vi "AutoShootRear.vi"() -> ()   [LabVIEW 2015]
uses:
  Typedef/IntakeControllerActions.ctl
  Typedef/IntakeControllerMsg.ctl
  ArmController/ArmController.lvlib
panel:
  in  "milliseconds to wait":u32=600
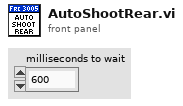
[diagram p1: front panel]
types:
  T1 = typedef "IntakeControllerMsg.ctl" = cluster{"Cmd":T2, "Data":variant}
  T2 = typedef "IntakeControllerActions.ctl" = enum16{"Wait on Intake Rear", "Wait on Angle Rear", "Go To Angle Rear", "Wait on Intake Front", "Wait on Angle Front", "Set Roller Front", "Set Roller Rear", "Go To Angle Front", "Wait ms"}
  T3 = cluster{"Down":dbl, "Pickup":dbl, "Shoot":dbl, "Turtle":dbl, "Intake Block":dbl, "Intake Transfer":dbl}
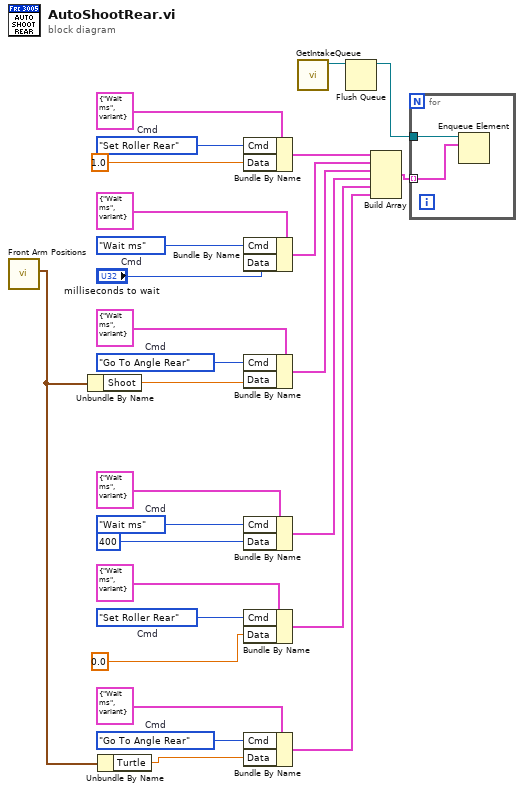
[diagram p0: block diagram]
diagram:
  w28 = IntakeControllerActions."Go To Angle Rear"  # Cmd
  w19 = IntakeControllerActions."Set Roller Rear"  # Cmd
  w23 = IntakeControllerActions."Wait ms"  # Cmd
  w16 = IntakeControllerActions."Go To Angle Rear"  # Cmd
  w11 = IntakeControllerActions."Wait ms"  # Cmd
  w8 = IntakeControllerActions."Set Roller Rear"  # Cmd
  n1 = call "Front Arm Positions.vi"() -> ("Rear Arm"=w1:T3)  [unwired: 10 in, 1 out]
  n2 = Unbundle By Name(w1) -> ("Shoot"=w2:dbl)
  n3 = Unbundle By Name(w1) -> ("Turtle"=w3:dbl)
  n4 = Bundle By Name(cluster=T1 {"Cmd"=enum."Wait ms", "Data"=variant(i32 50)} ("output cluster"), "Cmd"=w8, "Data"=1.0 ("Diffs")) -> (w10:T1)
  n5 = Bundle By Name(cluster=T1 {"Cmd"=enum."Wait ms", "Data"=variant(i32 50)} ("output cluster"), "Cmd"=w11, "Data"="milliseconds to wait") -> (w14:T1)
  n6 = Bundle By Name(cluster=T1 {"Cmd"=enum."Wait ms", "Data"=variant(i32 50)} ("output cluster"), "Cmd"=w16, "Data"=w2) -> (w17:T1)
  n7 = Bundle By Name(cluster=T1 {"Cmd"=enum."Wait ms", "Data"=variant(i32 50)} ("output cluster"), "Cmd"=w23, "Data"=u32 400 ("milliseconds to wait")) -> (w25:T1)
  n8 = Bundle By Name(cluster=T1 {"Cmd"=enum."Wait ms", "Data"=variant(i32 50)} ("output cluster"), "Cmd"=w19, "Data"=0.0 ("Diffs")) -> (w26:T1)
  n9 = Bundle By Name(cluster=T1 {"Cmd"=enum."Wait ms", "Data"=variant(i32 50)} ("output cluster"), "Cmd"=w28, "Data"=w3) -> (w5:T1)
  n10 = call "GetIntakeQueue.vi"() -> ("queue out"=w6:refnum<queue>)  [unwired: 11 in]
  n11 = Flush Queue(queue=w6) -> (queue out=w4:refnum<queue>)  [unwired: 1 in, 2 out]
  n12 = Build Array(w10, w14, w17, w25, w26, w5) -> (w18:T1[])
  n13 = for {
    tunnel: w4 -> [w30]
    tunnel: w18 -> [w29] mode=indexing
    n14 = Enqueue Element(queue=w30, element=w29) -> ()  [unwired: 2 in, 3 out]
  }
